vi "Readbundletree.vi"(8 "Error IN":errorcluster, 11 "HEKAdat.lvclass IN":refnum<class "HEKAdat.lvclass">) -> (0 "Error OUT":errorcluster, 3 "HEKAdat.lvclass OUT":refnum<class "HEKAdat.lvclass">)   [LabVIEW 2017, in "HEKAdat.lvclass"]
uses:
  HEKAdat.lvclass
  HEKAdat.lvclass/HEKAdat.ctl
panel:
  out "Seek":u32
  out "lvl_sizes":u32[](array[numeric])
  out "nlevels":u32
  out "magic":string
  out "End":u32[](array[numeric])
  out "Start":u32[](array[numeric])
  out "name":string[](array[string])
  out "nitems":u8
  out "time":dbl format="%.3f"
  out "Version":string
  out "Signature":string
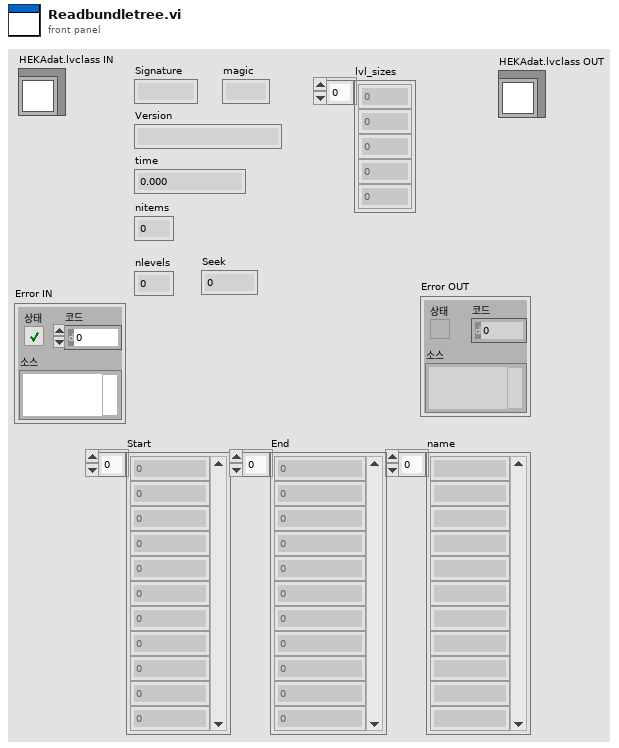
[diagram p1: front panel]
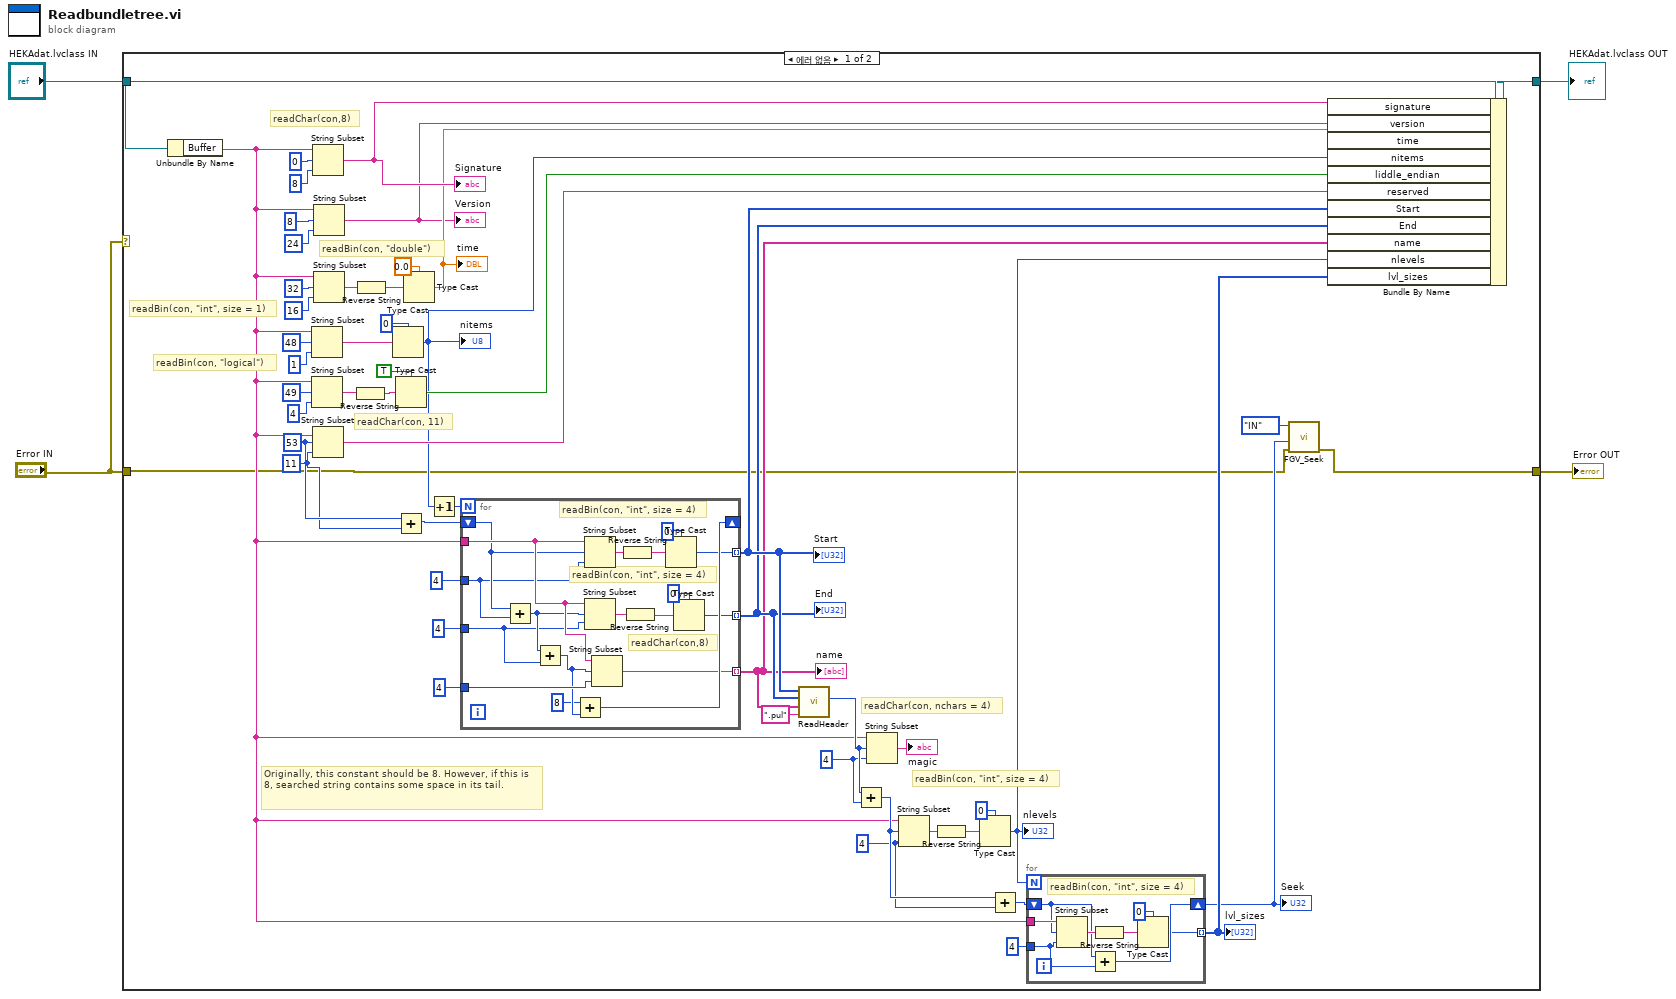
[diagram p0: block diagram]
diagram:
  n1 = case shown="에러 없음" "Error IN" {
    tunnel: "HEKAdat.lvclass IN" -> [w44 w86]
    tunnel: [w43 w86] -> w3
    tunnel: "Error IN" -> [w6 w85]
    tunnel: [w5 w85] -> w1
    frame No Error {
      w14 = 4 ("오프셋(0)")
      w17 = 4 ("오프셋(0)")
      w28 = 11 ("오프셋(0)")
      w29 = 53 ("오프셋(0)")
      # "readBin(con, \"int\", size = 4)"
      # "readChar(con, nchars = 4)"
      # "Originally, this constant should be 8. However, if this is 8, searched string contains some space in its tail."
      # "readChar(con, 11)"
      # "readBin(con, \"logical\")"
      # "readBin(con, \"int\", size = 1)"
      # "readBin(con, \"double\")"
      # "readChar(con,8)"
      n2 = Unbundle By Name(w44) -> ("Buffer"=w12:string)
      n3 = String Subset(string=w12, offset (0)=48 ("오프셋(0)"), length (rest)=1 ("오프셋(0)")) -> (substring=w40:string)
      n4 = String Subset(string=w12, offset (0)=49 ("오프셋(0)"), length (rest)=4 ("오프셋(0)")) -> (substring=w37:string)
      n5 = String Subset(string=w12, offset (0)=0 ("오프셋(0)"), length (rest)=8 ("오프셋(0)")) -> (substring=w46:string)
      "Signature" <- w46
      n6 = String Subset(string=w12, offset (0)=w29, length (rest)=w28) -> (substring=w35:string)
      n7 = String Subset(string=w12, offset (0)=8 ("오프셋(0)"), length (rest)=24 ("오프셋(0)")) -> (substring=w16:string)
      "Version" <- w16
      n8 = String Subset(string=w12, offset (0)=32 ("오프셋(0)"), length (rest)=16 ("오프셋(0)")) -> (substring=w51:string)
      n9 = Reverse String(1:w37) -> (0:w38:string)
      n10 = Reverse String(1:w51) -> (0:w50:string)
      n11 = Type Cast(type=u8 0 ("오프셋(0)"), x=w40) -> (*(type *) &x=w31:u8)
      "nitems" <- w31
      n12 = Type Cast(type=TRUE, x=w38) -> (*(type *) &x=w36:bool)
      n13 = Add(x=w29, y=w28) -> (x+y=w27:i32)
      n14 = Type Cast(type=0.0 ("오프셋(0)"), x=w50) -> (*(type *) &x=w45:dbl)
      "time" <- w45
      n15 = Increment(x=w31) -> (x+1=w30:u8)
      n16 = for {
        N: w30 -> [_]
        tunnel: w12 -> [w78]
        shift-right: [w71] -> _
        shift-left: w27 -> [w77]
        tunnel: 4 ("오프셋(0)") -> [w76]
        tunnel: 4 ("오프셋(0)") -> [w74]
        tunnel: 4 ("오프셋(0)") -> [w73]
        tunnel: [w70] -> w22 mode=indexing
        tunnel: [w69] -> w21 mode=indexing
        tunnel: [w68] -> w20 mode=indexing
        # "readChar(con,8)"
        # "readBin(con, \"int\", size = 4)"
        # "readBin(con, \"int\", size = 4)"
        n17 = Add(x=w77, y=w76) -> (x+y=w75:i32)
        n18 = Add(x=w75, y=w74) -> (x+y=w72:i32)
        n19 = Add(x=8, y=w72) -> (x+y=w71:i32)
        n20 = String Subset(string=w78, offset (0)=w77, length (rest)=w76) -> (substring=w80:string)
        n21 = String Subset(string=w78, offset (0)=w75, length (rest)=w74) -> (substring=w83:string)
        n22 = String Subset(string=w78, offset (0)=w72, length (rest)=w73) -> (substring=w68:string)
        n23 = Reverse String(1:w80) -> (0:w79:string)
        n24 = Reverse String(1:w83) -> (0:w84:string)
        n25 = Type Cast(type=u32 0, x=w79) -> (*(type *) &x=w70:u32)
        n26 = Type Cast(type=u32 0, x=w84) -> (*(type *) &x=w69:u32)
      }
      "Start" <- w22
      "End" <- w21
      "name" <- w20
      n27 = call "ReadHeader.vi"("name"=".pul", "[A] name"=w20, "End"=w21, "Start"=w22) -> ("Start"=w18:u32)  [unwired: 6 in, 1 out]
      n28 = Add(x=w18, y=w17) -> (x+y=w15:u32)
      n29 = String Subset(string=w12, offset (0)=w18, length (rest)=w17) -> (substring=→"magic":string)
      n30 = String Subset(string=w12, offset (0)=w15, length (rest)=w14) -> (substring=w24:string)
      n31 = Reverse String(1:w24) -> (0:w25:string)
      n32 = Type Cast(type=u32 0, x=w25) -> (*(type *) &x=w10:u32)
      "nlevels" <- w10
      n33 = Add(x=w15, y=w14) -> (x+y=w13:u32)
      n34 = for {
        N: w10 -> [_]
        shift-right: [w60] -> w8
        shift-left: w13 -> [w61]
        tunnel: w12 -> [w63]
        tunnel: 4 ("오프셋(0)") -> [w62]
        tunnel: [w59] -> w9 mode=indexing
        # "readBin(con, \"int\", size = 4)"
        n35 = String Subset(string=w63, offset (0)=w61, length (rest)=w62) -> (substring=w65:string)
        n36 = Add(x=w61, y=w62) -> (x+y=w60:u32)
        n37 = Reverse String(1:w65) -> (0:w64:string)
        n38 = Type Cast(type=u32 0, x=w64) -> (*(type *) &x=w59:u32)
      }
      "lvl_sizes" <- w9
      "Seek" <- w8
      n39 = call "FGV_Seek.vi"("Error IN"=w6, "Seek (con) IN"=w8, "IN or OUT"=enum16{"IN", "OUT"}."IN") -> ("Error OUT"=w5:errorcluster)  [unwired: 7 in, 1 out]
      n40 = Bundle By Name(cluster=w44, "signature"=w46, "version"=w16, "time"=w45, "nitems"=w31, "liddle_endian"=w36, "reserved"=w35, "Start"=w22, "End"=w21, "name"=w20, "nlevels"=w10, "lvl_sizes"=w9) -> (w43:refnum<class "HEKAdat.lvclass">)
    }
    frame Error {
    }
  }
  "HEKAdat.lvclass OUT" <- w3
  "Error OUT" <- w1
